vi "Generate Scan Coordinates.vi"(7 "Scan Pattern":T1(ring), 10 "Y Axis":T2, 11 "X Axis":T2) -> (1 "Array":cluster{"X":dbl, "Y":dbl}[](array[cluster]), 2 "Y Scale":dbl[](array[numeric]), 3 "X Scale":dbl[](array[numeric]))   [LabVIEW 2017]
uses:
  <vilib>/Analysis/1siggen.llb/Ramp Pattern by Samples.vi
  <vilib>/Analysis/NI_AALBase.lvlib
panel:
  out "XY Graph":cluster{"X":dbl, "Y":dbl}[](graph)
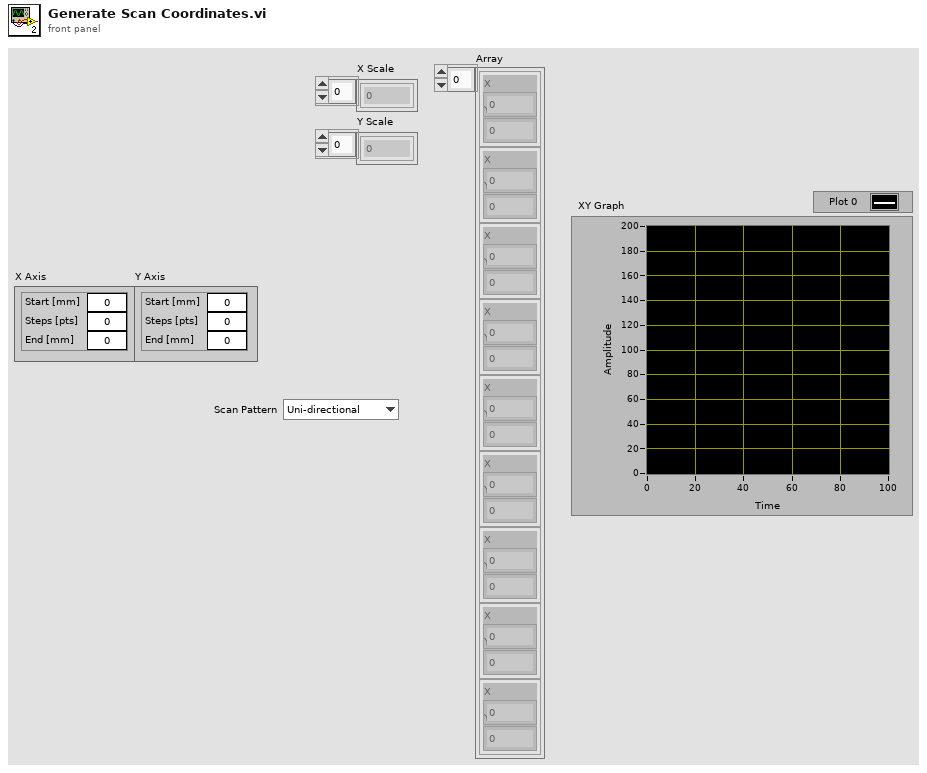
[diagram p1: front panel]
types:
  T1 = enum16{"Uni-directional", "Bi-Directional", "Spiral Out", "Spiral In"}
  T2 = cluster{"Start [mm]":dbl, "Steps [pts]":u16, "End [mm]":dbl}
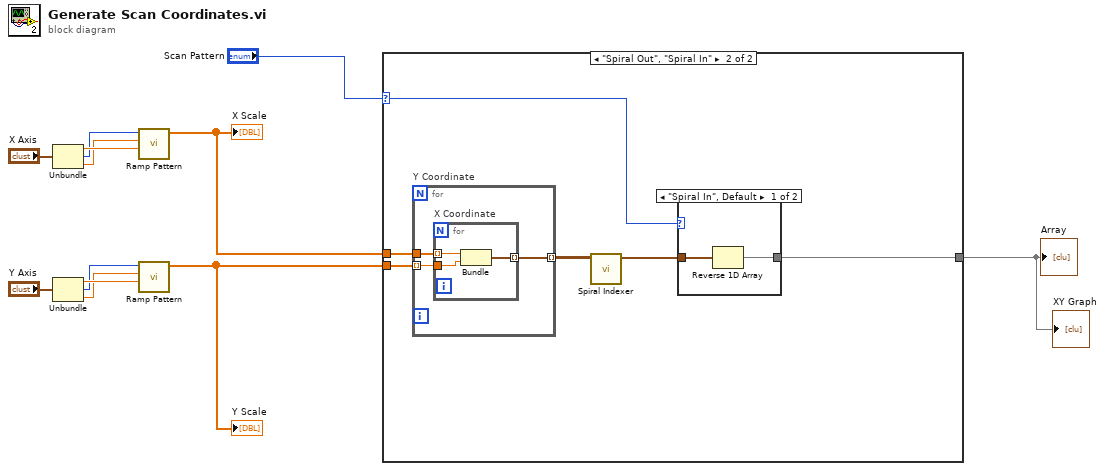
[diagram p0: block diagram]
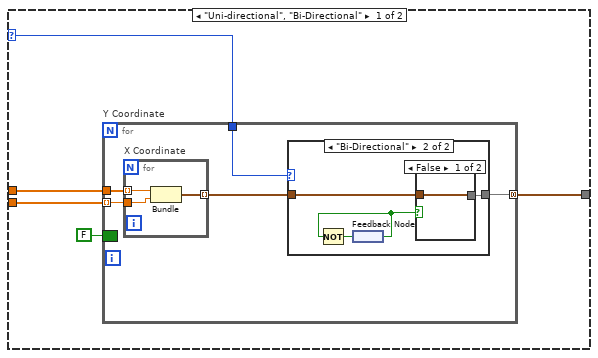
[diagram p2: hidden frame]
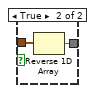
[diagram p4: hidden frame]
diagram:
  n1 = Unbundle("X Axis") -> ("Start [mm]"=w10:dbl, "Steps [pts]"=w9:u16, "End [mm]"=w8:dbl)
  n2 = Unbundle("Y Axis") -> ("Start [mm]"=w7:dbl, "Steps [pts]"=w5:u16, "End [mm]"=w6:dbl)
  n3 = call-poly <vilib>:"Ramp Pattern.vi"("start"=w10, "end"=w8, "samples"=w9) -> ("Ramp Pattern"=w4:dbl[])  [unwired: 7 in, 1 out]
  "X Scale" <- w4
  n4 = call-poly <vilib>:"Ramp Pattern.vi"("start"=w7, "end"=w6, "samples"=w5) -> ("Ramp Pattern"=w3:dbl[])  [unwired: 7 in, 1 out]
  "Y Scale" <- w3
  n5 = case shown="\"Spiral Out\", \"Spiral In\"" "Scan Pattern" {
    selector: "Scan Pattern" -> [w13 w36]
    tunnel: w4 -> [w17 w39]
    tunnel: w3 -> [w16 w38]
    tunnel: [w15 w35] -> w1
    frame "Uni-directional", "Bi-Directional" {
      n6 = for "Y Coordinate" {
        tunnel: w17 -> [w22]
        tunnel: w16 -> [w21] mode=indexing
        tunnel: [w18] -> w15 mode=concatenating
        tunnel: w13 -> [w20]
        border: FALSE -> [_]
        n7 = for "X Coordinate" {
          tunnel: w22 -> [w33] mode=indexing
          tunnel: w21 -> [w32]
          tunnel: [w31] -> w19 mode=indexing
          n8 = Bundle(w33, w32) -> (w31:cluster{dbl, dbl})  [unwired: 1 in]
        }
        n9 = case shown="\"Bi-Directional\"" w20 {
          tunnel: w19 -> [w23 w25]
          tunnel: [w23 w26] -> w18
          frame "Uni-directional", Default {
          }
          frame "Bi-Directional" {
            n10 = feedback #1() -> (w24:bool)
            n11 = Not(x=w24) -> (.not. x?=w27:bool)
            n12 = feedback-in #1(w27) -> ()
            n13 = case shown="False" w24 {
              tunnel: [w28 w30] -> w26
              tunnel: w25 -> [w28 w29]
              frame False {
              }
              frame True {
                n14 = Reverse 1D Array(array=w29) -> (reversed array=w30:cluster{dbl, dbl}[])
              }
            }
          }
        }
      }
    }
    frame "Spiral Out", "Spiral In" {
      n15 = for "Y Coordinate" {
        tunnel: w39 -> [w45]
        tunnel: w38 -> [w44] mode=indexing
        tunnel: [w43] -> w37 mode=indexing
        n16 = for "X Coordinate" {
          tunnel: w45 -> [w48] mode=indexing
          tunnel: w44 -> [w47]
          tunnel: [w46] -> w43 mode=indexing
          n17 = Bundle(w48, w47) -> (w46:cluster{dbl, dbl})  [unwired: 1 in]
        }
      }
      n18 = call "Spiral Indexer.vi"("Array 2"=w37) -> ("Array"=w34:cluster{dbl, dbl}[])  [unwired: 10 in]
      n19 = case shown="\"Spiral In\", Default" w36 {
        tunnel: [w40 w42] -> w35
        tunnel: w34 -> [w41 w42]
        frame "Spiral In", Default {
          n20 = Reverse 1D Array(array=w41) -> (reversed array=w40:cluster{dbl, dbl}[])
        }
        frame "Spiral Out" {
        }
      }
    }
  }
  "Array" <- w1
  "XY Graph" <- w1
